vi "写入NPLC.vi"(8 "error in (no error)":errorcluster caption="错误输入（无错误）", 10 "NPLC":dbl=10.0, 11 "Keithley 2000输入":refnum<class "Keithley 2000.lvclass">) -> (0 "error out":errorcluster caption="错误输出", 3 "Keithley 2000输出":refnum<class "Keithley 2000.lvclass">)   [LabVIEW 2020, in "DMM.lvlib" / "Keithley 2000.lvclass"]
uses:
  Keithley 2000.lvclass
  Keithley 2000.lvclass/Keithley 2000.ctl
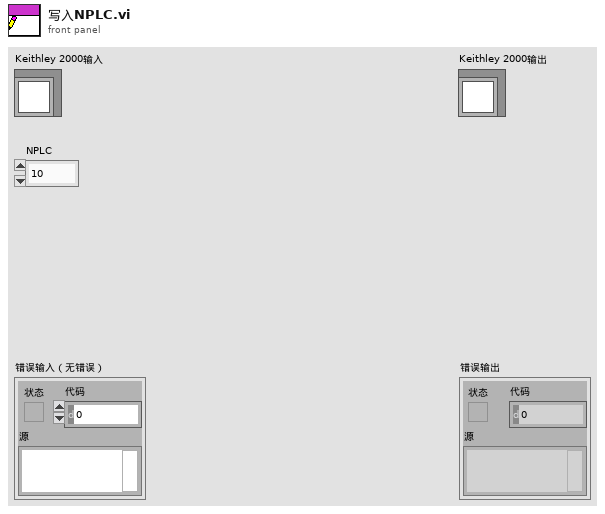
[diagram p1: front panel]
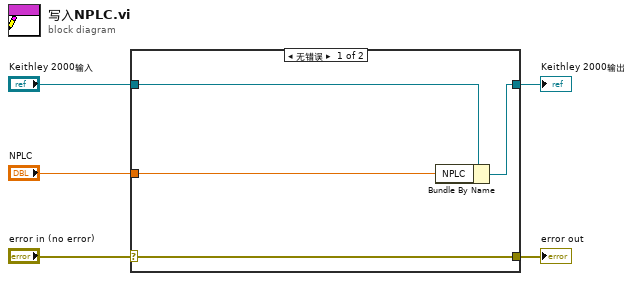
[diagram p0: block diagram]
diagram:
  n1 = case shown="无错误" "error in (no error)" {
    selector: "error in (no error)" -> [w9 w10]
    tunnel: [w9 w10] -> w4
    tunnel: [w7 w11] -> w2
    tunnel: "Keithley 2000输入" -> [w8 w11]
    tunnel: "NPLC" -> [w6 _]
    frame No Error {
      n2 = Bundle By Name(cluster=w8, "NPLC"=w6) -> (w7:refnum<class "Keithley 2000.lvclass">)
    }
    frame Error {
    }
  }
  "error out" <- w4
  "Keithley 2000输出" <- w2
